vi "Channel High Level Time.vi"(10 "Channel Index":i32, 11 "ASG Instr. A":T1 {"Time" format="%#.3p"}) -> (3 "Channel High Level Time (s)":ext=nan format="%#.5p")   [LabVIEW 2020]
uses:
  Labview Library/Libraries/HW_LMMR_ASG8100/LMMR ASG/ASG Instructions Data.ctl
  Labview Library/Libraries/HW_LMMR_ASG8100/LMMR ASG/Loop Config.ctl
  Labview Library/Libraries/HW_LMMR_ASG8100/LMMR ASG/Loop Code.ctl
  Labview Library/Libraries/HW_LMMR_ASG8100/LMMR ASG/Loop XControl.xctl
  Labview Library/Libraries/HW_LMMR_ASG8100/LMMR ASG/ASG Instructions XControl.xctl
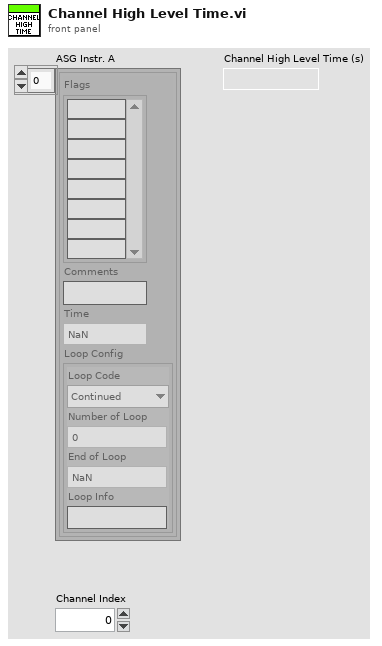
[diagram p1: front panel]
types:
  T1 = typedef "ASG Instructions XControl.xctl/ASG Instructions Data.ctl" = cluster{"Flags":bool[], "Comments":string, "Time":dbl, "Loop Config":T2}[]
  T2 = typedef "Loop XControl.xctl/Loop Config.ctl" = cluster{"Loop Code":T3, "Number of Loop":i32, "End of Loop":dbl, "Loop Info":string}
  T3 = typedef "Loop XControl.xctl/Loop Code.ctl" = enum16{"Continued", "Loop", "End Loop"}
  T4 = cluster{"Current Time":ext, "Current Instr Index":i32, "Loop Count":i32[], "Loop Index":i32[], "Loop Time":ext[]}
  T5 = cluster{"Flags":bool[], "Comments":string, "Time":dbl, "Loop Config":T2}
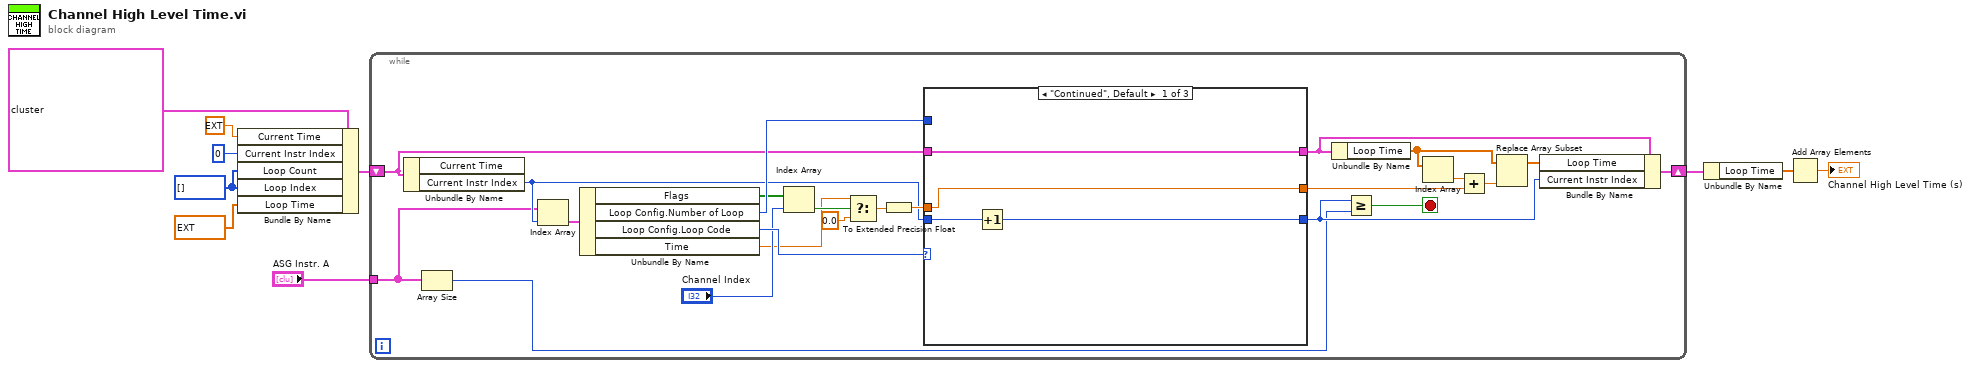
[diagram p0: block diagram]
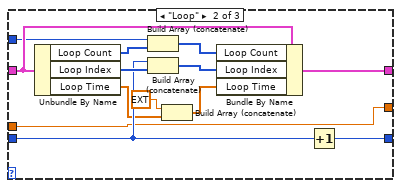
[diagram p2: hidden frame]
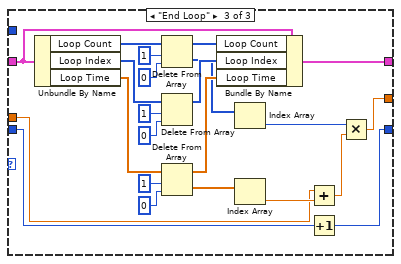
[diagram p3: hidden frame]
diagram:
  w7 = i32[] []
  n1 = Bundle By Name(cluster=T4 {"Current Time"=0.0, "Current Instr Index"=0, "Loop Count"=[], "Loop Index"=[], "Loop Time"=[]} ("Data"), "Current Time"=ext 0.0, "Current Instr Index"=0, "Loop Count"=w7, "Loop Index"=w7, "Loop Time"=ext[] [0.0]) -> (w5:T4)
  n2 = while {
    shift-right: [w33] -> w10
    shift-left: w5 -> [w29]
    tunnel: "ASG Instr. A" -> [w20]
    stop <- w17 stop-if-true
    n3 = Unbundle By Name(w29) -> ("Current Instr Index"=w26:i32)  [unwired: 1 out]
    n4 = Array Size(array=w20) -> (size(s)=w18:i32)
    n5 = Index Array(array=w20, index=w26) -> (element=w30:T5)
    n6 = Unbundle By Name(w30) -> ("Flags"=w16:bool[], "Loop Config.Number of Loop"=w31:i32, "Loop Config.Loop Code"=w32:T3, "Time"=w13:dbl)
    n7 = Index Array(array=w16, index="Channel Index") -> (element=w14:bool)
    n8 = Select(t=w13, s=w14, f=0.0) -> (s? t:f=w11:dbl)
    n9 = To Extended Precision Float(1:w11) -> (0:w28:ext)
    n10 = case shown="\"Continued\", Default" w32 {
      tunnel: w26 -> [w37 w42 w65]
      tunnel: [w36 w50 w64] -> w19
      tunnel: w31 -> [_ w45 _]
      tunnel: w29 -> [w35 w49 w73]
      tunnel: [w35 w48 w72] -> w25
      tunnel: w28 -> [w34 w39 w51]
      tunnel: [w34 w39 w53] -> w27
      frame "Continued", Default {
        n11 = Increment(x=w37) -> (x+1=w36:i32)
      }
      frame "Loop" {
        n12 = Unbundle By Name(w49) -> ("Loop Count"=w46:i32[], "Loop Index"=w43:i32[], "Loop Time"=w41:ext[])
        n13 = Build Array (concatenate)(w45, w46) -> (w44:i32[])
        n14 = Build Array (concatenate)(w42, w43) -> (w47:i32[])
        n15 = Build Array (concatenate)(ext 0.0, w41) -> (w40:ext[])
        n16 = Bundle By Name(cluster=w49, "Loop Count"=w44, "Loop Index"=w47, "Loop Time"=w40) -> (w48:T4)
        n17 = Increment(x=w42) -> (x+1=w50:i32)
      }
      frame "End Loop" {
        n18 = Unbundle By Name(w73) -> ("Loop Count"=w71:i32[], "Loop Index"=w70:i32[], "Loop Time"=w59:ext[])
        n19 = Delete From Array(array=w71, length=1, index=0) -> (deleted portion=w56:i32[], array with subset deleted=w63:i32[])
        n20 = Delete From Array(array=w70, length=1, index=0) -> (array with subset deleted=w62:i32[])  [unwired: 1 out]
        n21 = Delete From Array(array=w59, length=1, index=0) -> (deleted portion=w57:ext[], array with subset deleted=w58:ext[])
        n22 = Bundle By Name(cluster=w73, "Loop Count"=w63, "Loop Index"=w62, "Loop Time"=w58) -> (w72:T4)
        n23 = Index Array(array=w56) -> (element=w54:i32)  [unwired: 1 in]
        n24 = Index Array(array=w57) -> (element=w55:ext)  [unwired: 1 in]
        n25 = Add(x=w51, y=w55) -> (x+y=w52:ext)
        n26 = Increment(x=w65) -> (x+1=w64:i32)
        n27 = Multiply(x=w54, y=w52) -> (x*y=w53:ext)
      }
    }
    n28 = Unbundle By Name(w25) -> ("Loop Time"=w24:ext[])
    n29 = Greater Or Equal?(x=w19, y=w18) -> (x >= y?=w17:bool)
    n30 = Index Array(array=w24) -> (element=w23:ext)  [unwired: 1 in]
    n31 = Add(x=w23, y=w27) -> (x+y=w22:ext)
    n32 = Replace Array Subset(array=w24, new element=w22) -> (w21:ext[])  [unwired: 1 in]
    n33 = Bundle By Name(cluster=w25, "Loop Time"=w21, "Current Instr Index"=w19) -> (w33:T4)
  }
  n34 = Unbundle By Name(w10) -> ("Loop Time"=w3:ext[])
  n35 = Add Array Elements(numeric array=w3) -> (sum=→"Channel High Level Time (s)":ext)
